vi "dfd_Maxflat Filter Design Generate Table for M_NotZero.vi"(8 "H0":dbl, 9 "N":i32=2, 10 "M":i32=1, 11 "L":i32=3) -> (2 "fc":dbl)   [LabVIEW 2017, in "NI_DigFilter_Design.lvlib"]
doc: "Generates the table to keep the <B>L</B>, <B>M</B>, <B>N</B>, 0.5*min (angle frequency) and 0.5*mix (angle frequency) when <B>M</B>! = 0."
uses:
  <vilib>/addons/Digital Filter Design/NI_DigFilter_Design.lvlib
  <vilib>/addons/Digital Filter Design/NI_DigFilterLicensed.lvlib
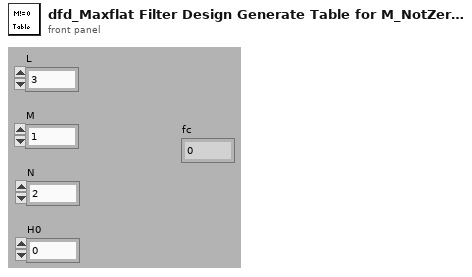
[diagram p1: front panel]
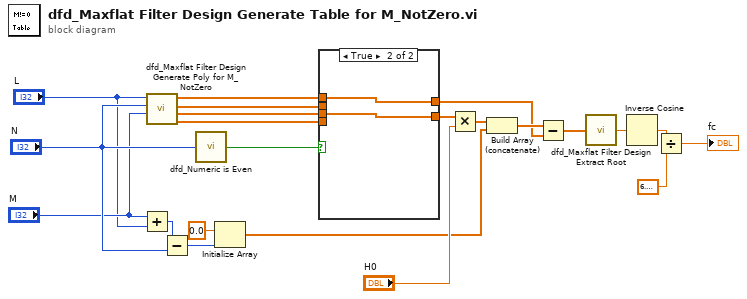
[diagram p0: block diagram]
diagram:
  n1 = Add(x="M", y="L") -> (x+y=w13:i32)
  n2 = call <vilib>:"dfd_Maxflat Filter Design Generate Poly for M_NotZero.vi"("M"="M", "N"="N", "L"="L") -> ("truncated APT"=w11:dbl[], "truncated APR-APT"=w10:dbl[], "APT"=w9:dbl[], "APR-APT"=w8:dbl[])  [unwired: 1 in, 4 out]
  n3 = Subtract(x=w13, y="N") -> (x-y=w14:i32)
  n4 = call <vilib>:"dfd_Numeric is Even.vi"("N"="N") -> ("even ?"=w16:bool)
  n5 = Initialize Array(0.0 ("element"), w14) -> (w4:dbl[])
  n6 = case shown="True" w16 {
    tunnel: w9 -> [w24 _]
    tunnel: w10 -> [_ w25]
    tunnel: w11 -> [w23 _]
    tunnel: w8 -> [_ w26]
    tunnel: [w24 w26] -> w2
    tunnel: [w23 w25] -> w7
    frame False {
    }
    frame True {
    }
  }
  n7 = Multiply(x=w7, y="H0") -> (x*y=w5:dbl[])
  n8 = Build Array (concatenate)(w5, w4) -> (w3:dbl[])
  n9 = Subtract(x=w3, y=w2) -> (x-y=w1:dbl[])
  n10 = call <vilib>:"dfd_Maxflat Filter Design Extract Root.vi"("input polynomial"=w1) -> ("extracted root"=w19:dbl)
  n11 = Inverse Cosine(1:w19) -> (0:w17:dbl)
  n12 = Divide(x=w17, y=6.283185307179586) -> (x/y=→"fc":dbl)
